vi "normalise_QPD_signal.vi"(9 "SUM in":waveform(dbl), 10 "BT in":waveform(dbl), 11 "LR in":waveform(dbl)) -> (1 "SUM out":waveform(dbl), 2 "BT out":waveform(dbl), 3 "LR out":waveform(dbl))   [LabVIEW 2019]
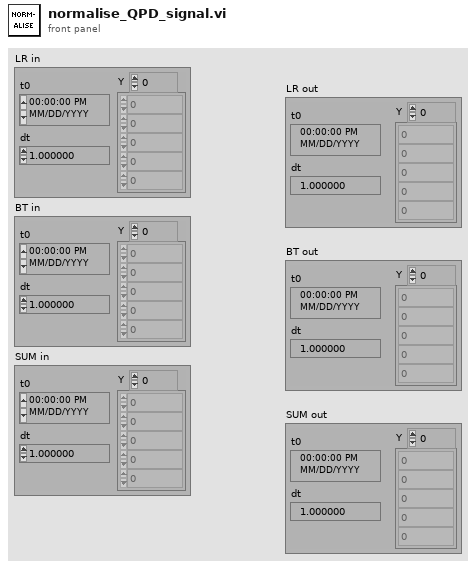
[diagram p1: front panel]
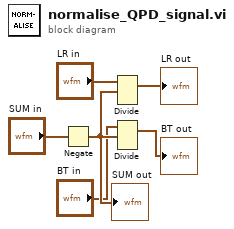
[diagram p0: block diagram]
diagram:
  n1 = Negate(x="SUM in") -> (-x=w4:waveform(dbl))
  "SUM out" <- w4
  n2 = Divide(1:w4, 2:"LR in") -> (0:→"LR out":waveform(dbl))  [unwired: 1 in, 1 out]
  n3 = Divide(1:w4, 2:"BT in") -> (0:→"BT out":waveform(dbl))  [unwired: 1 in, 1 out]
